vi "ReAnchor Steps POLY.vi"   [LabVIEW 2020, in "BetterDragAndDrop.lvlib" / "BetterTreeHandle.lvclass"]
uses:
  BetterTreeHandle/BetterTreeHandle.lvclass
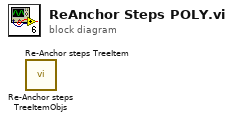
[diagram p0: block diagram]
diagram:
  n1 = call "Re-Anchor steps TreeItemObjs.vi"() -> ()  [unwired: 11 in, 1 out]
  n2 = call "Re-Anchor steps TreeItem.vi"() -> ()  [unwired: 11 in, 1 out]
